vi "MDAQ_Parse_Spectrum.vi"(8 "error in":errorcluster, 9 "?":T1 {"GATESTOP" format="%04x"; "GATESTRT" format="%04x"; "AMPLITUDE" format="%04x"; "M_CYCLES" format="%04x"; "N_CYCLES" format="%04x"; "STEP" format="%04x"; "BASE" format="%04x"; "CHAN" format="%04x"}, 10 "input buffer":string) -> (0 "error out":errorcluster, 1 "output cluster":T1 {"GATESTOP" format="%04x"; "GATESTRT" format="%04x"; "AMPLITUDE" format="%04x"; "M_CYCLES" format="%04x"; "N_CYCLES" format="%04x"; "STEP" format="%04x"; "BASE" format="%04x"; "CHAN" format="%04x"}, 2 "Array":u32[](array[numeric]))   [LabVIEW 2021]
uses:
  Status_Cluster.ctl
  <vilib>/regexp/Match Regular Expression.xnode
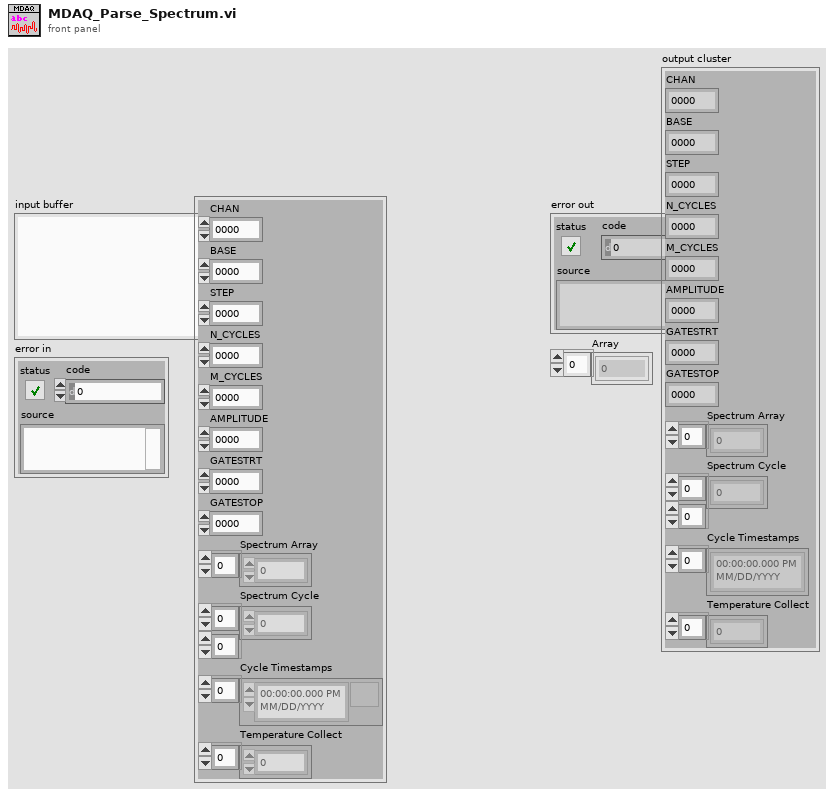
[diagram p1: front panel]
types:
  T1 = typedef "Status_Cluster.ctl" = cluster{"CHAN":u32, "BASE":u32, "STEP":u32, "N_CYCLES":u32, "M_CYCLES":u32, "AMPLITUDE":u32, "GATESTRT":u32, "GATESTOP":u32, "Spectrum Array":u32[], "Spectrum Cycle":u32[][], "Cycle Timestamps":timestamp[], "Temperature Collect":dbl[]}
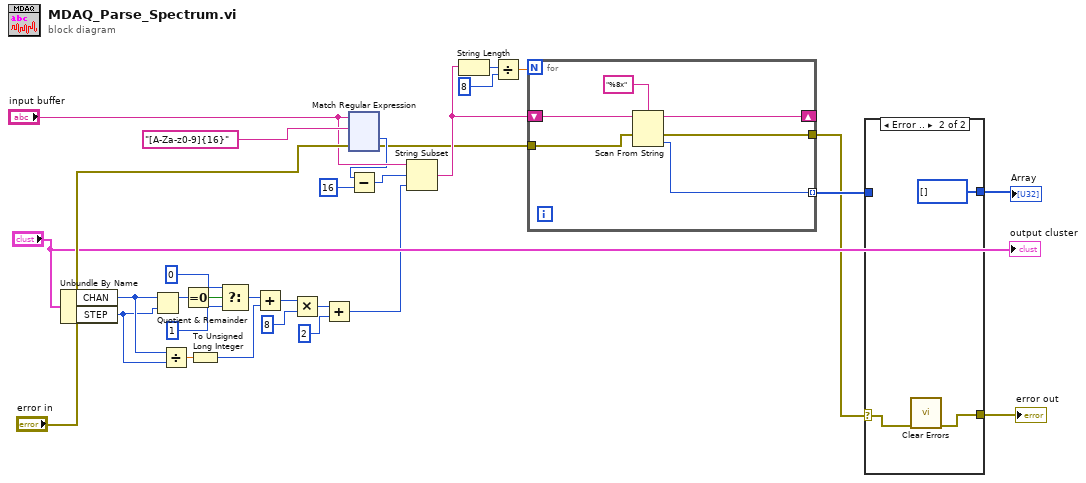
[diagram p0: block diagram]
diagram:
  n1 = Unbundle By Name("?") -> ("CHAN"=w24:u32, "STEP"=w23:u32)
  n2 = Quotient & Remainder(x=w24, y=w23) -> (x-y*floor(x/y)=w28:u32)  [unwired: 1 out]
  n3 = Divide(x=w24, y=w23) -> (x/y=w21:dbl)
  n4 = Equal To 0?(x=w28) -> (x = 0?=w27:bool)
  n5 = To Unsigned Long Integer(number=w21) -> (unsigned 32bit integer=w20:u32)
  n6 = Select(t=u32 0, s=w27, f=u32 1) -> (s? t:f=w22:u32)
  n7 = Add(x=w22, y=w20) -> (x+y=w19:u32)
  n8 = Multiply(x=w19, y=u32 8) -> (x*y=w17:u32)
  n9 = Add(x=w17, y=u32 2) -> (x+y=w10:u32)
  n10 = xnode "Match Regular Expression"("input string"="input buffer", "regular expression"="[A-Za-z0-9]{16}", "error in"="error in") -> ("offset past match"=w13:i32, "error out"=w5:errorcluster)  [unwired: 3 in, 3 out]
  n11 = Subtract(x=w13, y=16) -> (x-y=w11:i32)
  n12 = String Subset(string="input buffer", offset (0)=w11, length (rest)=w10) -> (substring=w6:string)
  n13 = String Length(string=w6) -> (length=w9:i32)
  n14 = Divide(x=w9, y=8) -> (x/y=w7:dbl)
  n15 = for {
    N: w7 -> [_]
    shift-right: [w34] -> _
    shift-left: w6 -> [w36]
    tunnel: w5 -> [w33]
    tunnel: [w32] -> w2
    tunnel: [w31] -> w4 mode=indexing
    n16 = Scan From String(format string="%8x", input string=w36, error in=w33) -> (remaining string=w34:string, error out=w32:errorcluster, output 1=w31:u32)  [unwired: 2 in, 1 out]
  }
  n17 = case shown="Error .." w2 {
    selector: w2 -> [w37 w40]
    tunnel: w4 -> [w38 _]
    tunnel: [w38 u32[] []] -> w3
    tunnel: [w37 w39] -> w1
    frame No Error {
    }
    frame Error {
      n18 = call <vilib>:"Clear Errors.vi"("error in (no error)"=w40) -> ("error out"=w39:errorcluster)  [unwired: 5 in, 1 out]
    }
  }
  "error out" <- w1
  "Array" <- w3
  "output cluster" <- "?"
